vi "localizador.vi"(9 "Orden":T2(array[ring])=[enum."espejos", enum."voltaje", enum."polarizador", enum."potenciometro ", enum."CCD"]) -> (1 "Tipo de Medición":T1(ring), 2 "Enum":T3(ring))   [LabVIEW 2016]
panel:
  out "subarray":T2(array[ring])
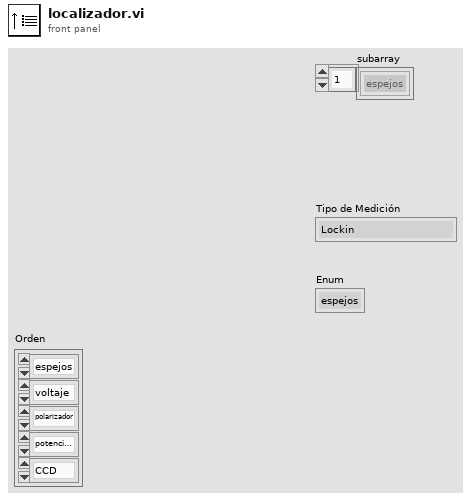
[diagram p1: front panel]
types:
  T1 = enum16{"Lockin", "Lockin-potenciometro", "Potenciometro"}
  T2 = enum16{"espejos", "polarizador", "voltaje", "potenciometro ", "CCD", "lockin", "laser", "ninguno"}[]
  T3 = enum16{"espejos", "polarizador", "voltaje", "potenciometro ", "CCD", "lockin", "laser", "ninguno"}
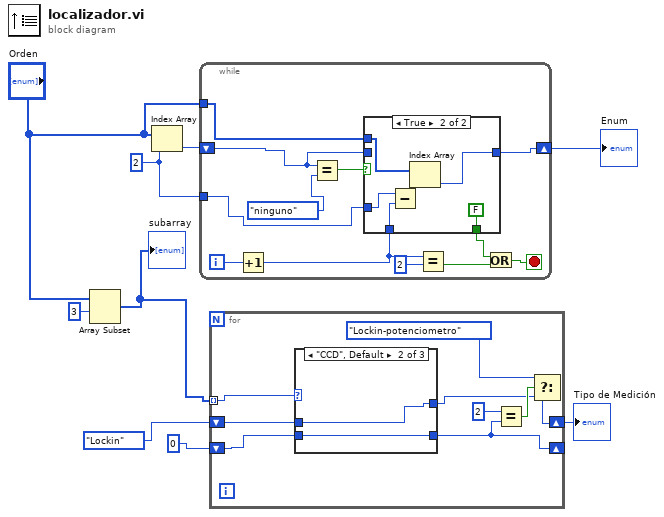
[diagram p0: block diagram]
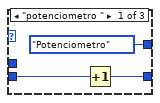
[diagram p2: hidden frame]
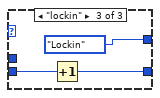
[diagram p3: hidden frame]
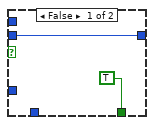
[diagram p4: hidden frame]
diagram:
  w7 = 2 ("index")
  n1 = Array Subset(array="Orden", index=3) -> (w4:T2)  [unwired: 1 in]
  "subarray" <- w4
  n2 = Index Array(array="Orden", index=w7) -> (element=w9:T3)
  n3 = while {
    shift-right: [w16] -> w8
    shift-left: w9 -> [w15]
    tunnel: w7 -> [w19]
    tunnel: "Orden" -> [w17]
    i -> [w18]
    stop <- w14 stop-if-true
    n4 = Increment(x=w18) -> (x+1=w13:i32)
    n5 = Equal?(x=w15, y=T3."ninguno" ("Enum")) -> (x = y?=w20:bool)
    n6 = case shown="True" w20 {
      tunnel: [TRUE FALSE] -> w11
      tunnel: w19 -> [_ w28]
      tunnel: w17 -> [_ w29]
      tunnel: w13 -> [_ w27]
      tunnel: [w22 w25] -> w16
      tunnel: w15 -> [w22 _]
      frame False {
      }
      frame True {
        n7 = Subtract(x=w28, y=w27) -> (x-y=w26:i32)
        n8 = Index Array(array=w29, index=w26) -> (element=w25:T3)
      }
    }
    n9 = Equal?(x=w13, y=2) -> (x = y?=w10:bool)
    n10 = Or(x=w11, y=w10) -> (x .or. y?=w14:bool)
  }
  "Enum" <- w8
  n11 = for {
    tunnel: w4 -> [w38] mode=indexing
    shift-right: [w33] -> w1
    shift-left: T1."Lockin" ("Tipo de Medición") -> [w36]
    shift-right: [w35] -> _
    shift-left: 0 -> [w37]
    n12 = case shown="\"CCD\", Default" w38 {
      tunnel: w37 -> [w39 w43 w46]
      tunnel: [w40 w43 w45] -> w35
      tunnel: [T1."Potenciometro" ("Tipo de Medición") w42 T1."Lockin" ("Tipo de Medición")] -> w31
      tunnel: w36 -> [_ w42 _]
      frame "potenciometro " {
        n13 = Increment(x=w39) -> (x+1=w40:i32)
      }
      frame "CCD", Default {
      }
      frame "lockin" {
        n14 = Increment(x=w46) -> (x+1=w45:i32)
      }
    }
    n15 = Equal?(x=2, y=w35) -> (x = y?=w32:bool)
    n16 = Select(t=T1."Lockin-potenciometro", s=w32, f=w31) -> (s? t:f=w33:T1)
  }
  "Tipo de Medición" <- w1
